vi "FPGA_ADC_send_orders.vi"(5 "option":T3(ring), 6 "Trigger":T1={"mode"=enum."RT", "source"=1, "edge"=enum."falling"}, 7 "FPGA VI Reference In":T2, 8 "sample count":u32, 9 "channel config":u16, 10 "avg per point":u16, 11 "40MHz divider":u32) -> (1 "order out":u64, 2 "FPGA VI Reference Out":T2)   [LabVIEW 2013]
uses:
  fpga-bitfile-ref.ctl
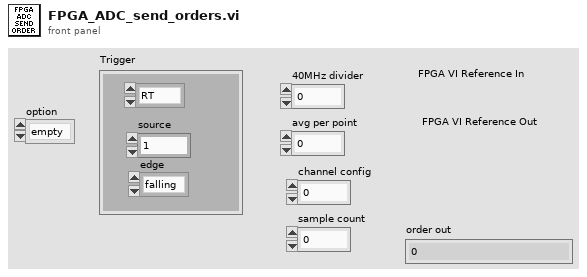
[diagram p1: front panel]
types:
  T1 = cluster{"mode":enum8{"ramp", "RT"}, "source":u8, "edge":enum8{"falling", "rising", "both"}}
  T2 = typedef "fpga-bitfile-ref.ctl" = refnum<k20>
  T3 = enum16{"empty", "stop", "start", "sampling rate", "trigger", "sample count", "reset channels", "add channel", "avg per point", "manual trigger"}
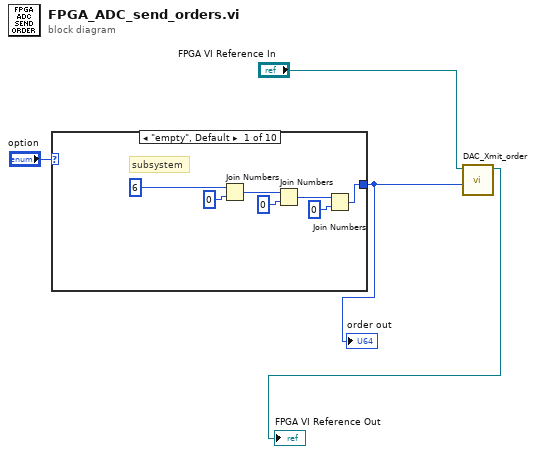
[diagram p0: block diagram]
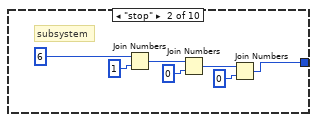
[diagram p2: hidden frame]
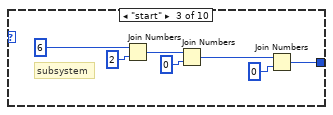
[diagram p3: hidden frame]
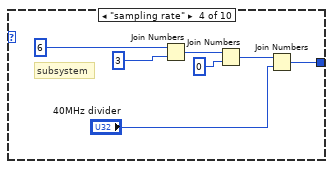
[diagram p4: hidden frame]
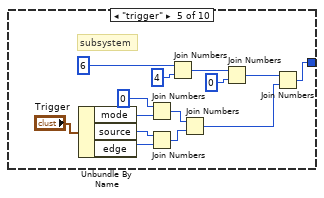
[diagram p5: hidden frame]
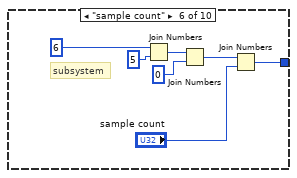
[diagram p6: hidden frame]
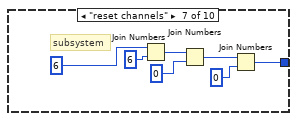
[diagram p7: hidden frame]
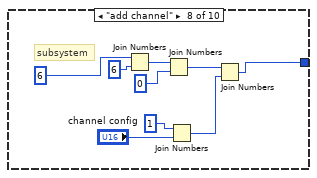
[diagram p8: hidden frame]
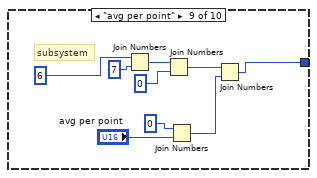
[diagram p9: hidden frame]
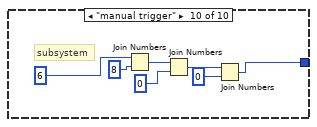
[diagram p10: hidden frame]
diagram:
  n1 = case shown="\"empty\", Default" "option" {
    tunnel: [w5 w12 w20 w28 w36 w48 w56 w64 w73 w80] -> w4
    frame "empty", Default {
      # "subsystem"
      n2 = Join Numbers(hi=u8 6, lo=u8 0) -> ((hi.lo)=w11:u16)
      n3 = Join Numbers(hi=w11, lo=u16 0) -> ((hi.lo)=w9:u32)
      n4 = Join Numbers(hi=w9, lo=u32 0) -> ((hi.lo)=w5:u64)
    }
    frame "stop" {
      # "subsystem"
      n5 = Join Numbers(hi=u8 6, lo=u8 1) -> ((hi.lo)=w18:u16)
      n6 = Join Numbers(hi=w18, lo=u16 0) -> ((hi.lo)=w16:u32)
      n7 = Join Numbers(hi=w16, lo=u32 0) -> ((hi.lo)=w12:u64)
    }
    frame "start" {
      # "subsystem"
      n8 = Join Numbers(hi=u8 6, lo=u8 2) -> ((hi.lo)=w25:u16)
      n9 = Join Numbers(hi=w25, lo=u16 0) -> ((hi.lo)=w23:u32)
      n10 = Join Numbers(hi=w23, lo=u32 0) -> ((hi.lo)=w20:u64)
    }
    frame "sampling rate" {
      # "subsystem"
      n11 = Join Numbers(hi=u8 6, lo=u8 3) -> ((hi.lo)=w32:u16)
      n12 = Join Numbers(hi=w32, lo=u16 0) -> ((hi.lo)=w30:u32)
      n13 = Join Numbers(hi=w30, lo="40MHz divider") -> ((hi.lo)=w28:u64)
    }
    frame "trigger" {
      # "subsystem"
      n14 = Unbundle By Name("Trigger") -> ("mode"=w39:enum8{"ramp", "RT"}, "source"=w34:u8, "edge"=w33:enum8{"falling", "rising", "both"})
      n15 = Join Numbers(hi=u8 0 ("lo"), lo=w39) -> ((hi.lo)=w38:u16)
      n16 = Join Numbers(hi=w34, lo=w33) -> ((hi.lo)=w37:u16)
      n17 = Join Numbers(hi=u8 6, lo=u8 4) -> ((hi.lo)=w46:u16)
      n18 = Join Numbers(hi=w38, lo=w37) -> ((hi.lo)=w35:u32)
      n19 = Join Numbers(hi=w46, lo=u16 0) -> ((hi.lo)=w44:u32)
      n20 = Join Numbers(hi=w44, lo=w35) -> ((hi.lo)=w36:u64)
    }
    frame "sample count" {
      # "subsystem"
      n21 = Join Numbers(hi=u8 6, lo=u8 5) -> ((hi.lo)=w53:u16)
      n22 = Join Numbers(hi=w53, lo=u16 0) -> ((hi.lo)=w51:u32)
      n23 = Join Numbers(hi=w51, lo="sample count") -> ((hi.lo)=w48:u64)
    }
    frame "reset channels" {
      # "subsystem"
      n24 = Join Numbers(hi=u8 6, lo=u8 6) -> ((hi.lo)=w60:u16)
      n25 = Join Numbers(hi=w60, lo=u16 0) -> ((hi.lo)=w58:u32)
      n26 = Join Numbers(hi=w58, lo=u32 0) -> ((hi.lo)=w56:u64)
    }
    frame "add channel" {
      # "subsystem"
      n27 = Join Numbers(hi=u8 6, lo=u8 6) -> ((hi.lo)=w65:u16)
      n28 = Join Numbers(hi=w65, lo=u16 0) -> ((hi.lo)=w67:u32)
      n29 = Join Numbers(hi=u16 1, lo="channel config") -> ((hi.lo)=w63:u32)
      n30 = Join Numbers(hi=w67, lo=w63) -> ((hi.lo)=w64:u64)
    }
    frame "avg per point" {
      # "subsystem"
      n31 = Join Numbers(hi=u8 6, lo=u8 7) -> ((hi.lo)=w74:u16)
      n32 = Join Numbers(hi=w74, lo=u16 0) -> ((hi.lo)=w76:u32)
      n33 = Join Numbers(hi=u16 0, lo="avg per point") -> ((hi.lo)=w72:u32)
      n34 = Join Numbers(hi=w76, lo=w72) -> ((hi.lo)=w73:u64)
    }
    frame "manual trigger" {
      # "subsystem"
      n35 = Join Numbers(hi=u8 6, lo=u8 8) -> ((hi.lo)=w81:u16)
      n36 = Join Numbers(hi=w81, lo=u16 0) -> ((hi.lo)=w83:u32)
      n37 = Join Numbers(hi=w83, lo=u32 0) -> ((hi.lo)=w80:u64)
    }
  }
  "order out" <- w4
  n38 = call "DAC_Xmit_order.vi"("Order in"=w4, "FPGA VI Reference In"="FPGA VI Reference In") -> ("FPGA VI Reference Out"=→"FPGA VI Reference Out":T2)  [unwired: 9 out]
